vi "TranslateLabel.vi"(0 "reference":refnum<class "SegmentedLineEdge.lvclass">, 1 "dx":dbl format="%.2f", 2 "dy":dbl format="%.2f", 3 "Label(Mid)":enum16{"Mid"}(ring), 5 "error in (no error)":errorcluster) -> (14 "reference out":refnum<class "SegmentedLineEdge.lvclass">, 19 "error out":errorcluster)   [LabVIEW 2016, in "SegmentedLineEdge.lvclass"]
doc: "Translate"
uses:
  <resource>/Framework/Providers/Open_GDS/UML/SegmentedLineEdge_class/SegmentedLineEdge.lvclass
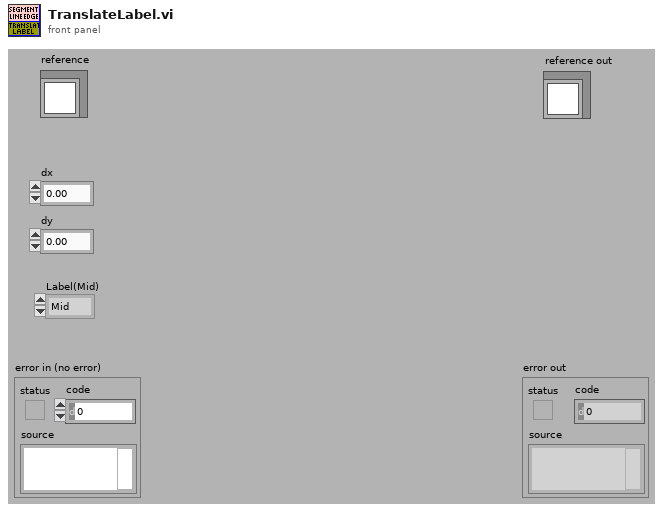
[diagram p1: front panel]
types:
  T1 = typedef "SegmentedLineEdge.lvclass/ObjectAttributes.ctl" = cluster{"lineStyle":refnum<class "LineStyle.lvclass">, "startArrowHead":refnum<class "ArrowHead.lvclass">, "endArrowHead":refnum<class "ArrowHead.lvclass">, "startLabel":string, "midLabel":string, "endLabel":string, "MidLabelOffset":T2, "SplitWire":bool}
  T2 = typedef "Point Point2D.ctl" = cluster{"x":dbl, "y":dbl}
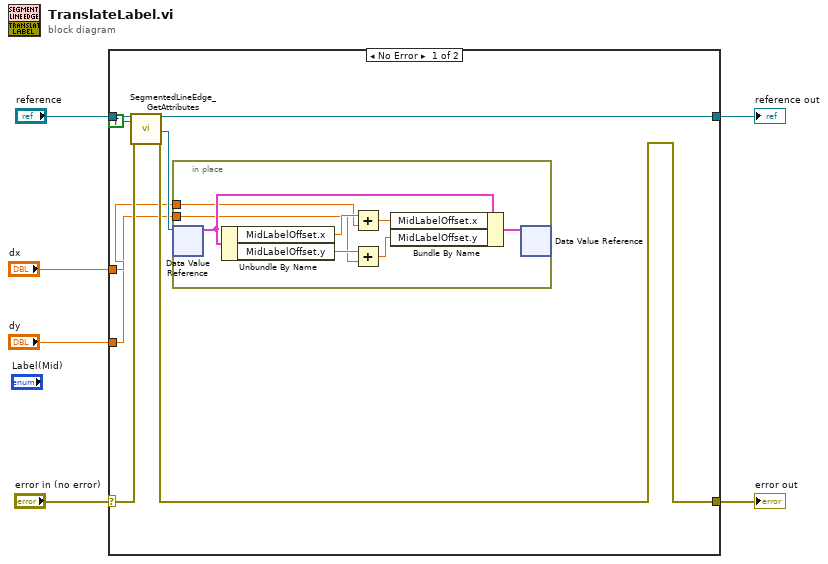
[diagram p0: block diagram]
diagram:
  n1 = case shown="No Error" "error in (no error)" {
    selector: "error in (no error)" -> [w14 w23]
    tunnel: "reference" -> [w13 w24]
    tunnel: [w12 w23] -> w4
    tunnel: [w11 w24] -> w3
    tunnel: "dx" -> [w8 _]
    tunnel: "dy" -> [w7 _]
    frame No Error {
      n2 = call <resource>:"SegmentedLineEdge_GetAttributes.vi"("reference in"=w13, "OnlyGetDvrReference(False)"=TRUE, "error in (no error)"=w14) -> ("reference out"=w11:refnum<class "SegmentedLineEdge.lvclass">, "DataRef"=w9:refnum<data-value>, "error out"=w12:errorcluster)  [unwired: 13 in, 1 out]
      n3 = in-place {
        in-place-border: w8 -> [w16]
        in-place-border: w7 -> [w15]
        n4 = in-place-dvr #1(w9) -> (w22:T1)  [unwired: 1 out]
        n5 = Unbundle By Name(w22) -> ("MidLabelOffset.x"=w18:dbl, "MidLabelOffset.y"=w17:dbl)
        n6 = Add(x=w18, y=w16) -> (x+y=w21:dbl)
        n7 = Add(x=w17, y=w15) -> (x+y=w20:dbl)
        n8 = Bundle By Name(cluster=w22, "MidLabelOffset.x"=w21, "MidLabelOffset.y"=w20) -> (w19:T1)
        n9 = in-place-dvr #1(w19) -> ()  [unwired: 2 out]
      }
    }
    frame Error {
    }
  }
  "reference out" <- w3
  "error out" <- w4
